vi "Functions_Load All.vi"(0 "scripts manager in":refnum<class "scripts manager.lvclass">, 5 "Function Path":path, 7 "Output Terminal":refnum<class "Output Terminal.lvclass">, 9 "RT Variables":refnum<class "RT Variables.lvclass">, 11 "error in (no error)":errorcluster) -> (4 "scripts manager out":refnum<class "scripts manager.lvclass">, 15 "error out":errorcluster)   [LabVIEW 2019, in "LSL.lvlib" / "scripts manager.lvclass"]
uses:
  scripts manager.lvclass
  output terminal/Base/Output Terminal.lvclass
  variables/RT Variables/RT Variables.lvclass
  scripts manager.lvclass/scripts manager.ctl
  functions/functionsbase/functionbase.lvclass
  functions/functionsbase/functionbase.lvclass/functionbase.ctl
  functions/functionsbase/properties/Write Output Terminal.vi
  functions/functionsbase/properties/Write RT Variables.vi
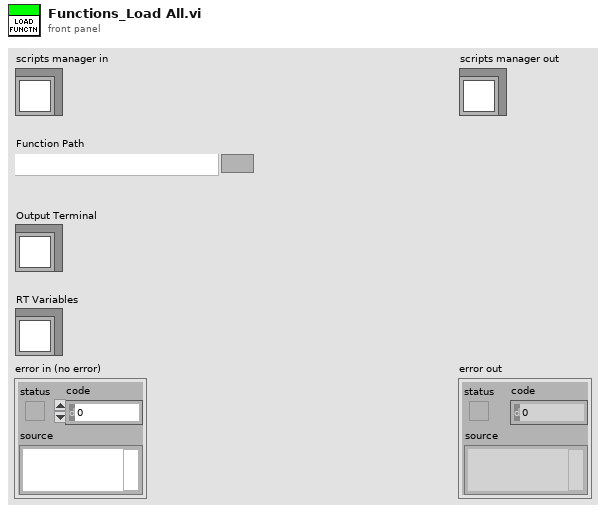
[diagram p1: front panel]
types:
  T1 = typedef "Scan Syntax Format.ctl" = cluster{"Format String":string, "Variable#":i32, "Variables Name":string[]}
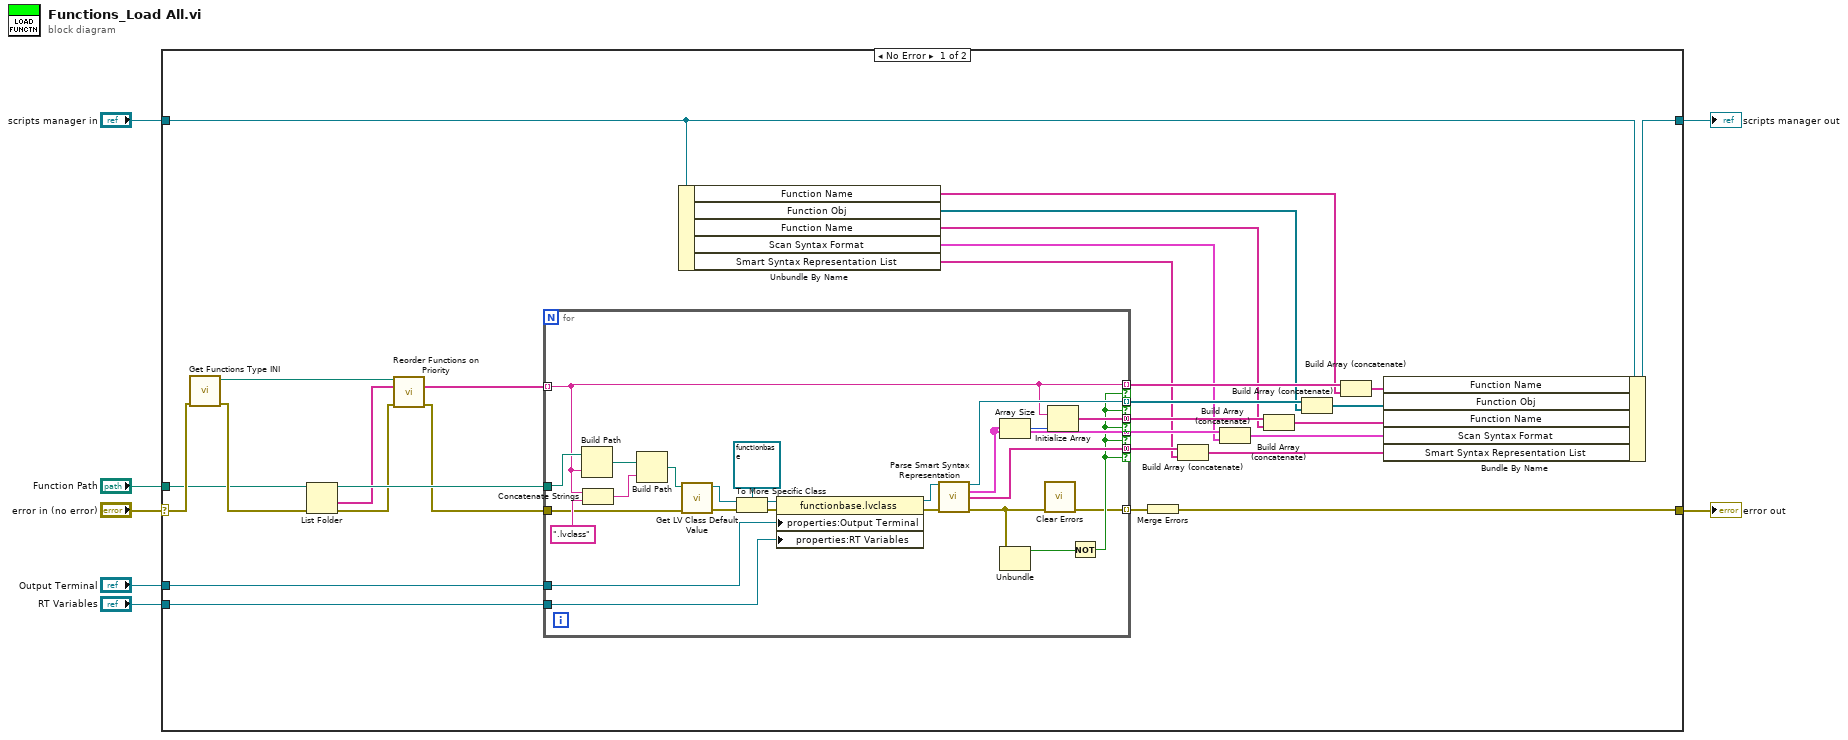
[diagram p0: block diagram]
diagram:
  n1 = case shown="No Error" "error in (no error)" {
    selector: "error in (no error)" -> [w22 w64]
    tunnel: [w31 w64] -> w6
    tunnel: [w32 w63] -> w4
    tunnel: "scripts manager in" -> [w19 w63]
    tunnel: "Output Terminal" -> [w28 _]
    tunnel: "RT Variables" -> [w27 _]
    tunnel: "Function Path" -> [w8 _]
    frame No Error {
      n2 = call "Get Functions Type INI.vi"("error in"=w22) -> ("error out"=w21:errorcluster, "Function Config INI"=w20:path)  [unwired: 9 in]
      n3 = List Folder(path=w8, error in=w21) -> (path out=w37:path, folder names=w23:string[], error out=w26:errorcluster)  [unwired: 2 in, 1 out]
      n4 = call "Reorder Functions on Priority.vi"("config path"=w20, "Function List"=w23, "error in (no error)"=w26) -> ("Function List out"=w24:string[], "error out"=w25:errorcluster)  [unwired: 11 in]
      n5 = for {
        tunnel: w25 -> [w57]
        tunnel: w24 -> [w48] mode=indexing
        tunnel: w37 -> [w62]
        tunnel: [w38] -> w36 mode=indexing
        tunnel: [w51] -> w29 mode=indexing if=w45
        tunnel: [w48] -> w30 mode=indexing if=w45
        tunnel: [w50] -> w35 mode=concatenating if=w45
        tunnel: [w47] -> w33 mode=concatenating if=w45
        tunnel: [w46] -> w34 mode=concatenating if=w45
        tunnel: w28 -> [w40]
        tunnel: w27 -> [w39]
        n6 = Build Path(base path=w62, name or relative path=w48) -> (appended path=w61:path)
        n7 = Concatenate Strings(w48, ".lvclass" ("string")) -> (w59:string)
        n8 = Build Path(base path=w61, name or relative path=w59) -> (appended path=w58:path)
        n9 = call <vilib>:"Get LV Class Default Value.vi"("error in (no error)"=w57, "class path"=w58) -> ("error out"=w56:errorcluster, "object"=w55:refnum<class>)  [unwired: 8 in]
        n10 = To More Specific Class(target class=refnum<class "functionbase.lvclass"> refnum ("functionbase.lvclass"), reference=w55, error in=w56) -> (specific class reference=w42:refnum<class "functionbase.lvclass">, error out=w44:errorcluster)
        n11 = property class="functionbase.lvclass"(reference=w42, error in=w44, "properties:Output Terminal"=w40, "properties:RT Variables"=w39) -> (reference out=w41:refnum<class "functionbase.lvclass">, error out=w43:errorcluster)
        n12 = call-dynamic "Parse Smart Syntax Representation.vi"("functionbase in"=w41, "error in (no error)"=w43) -> ("functionbase out"=w51:refnum<class "functionbase.lvclass">, "Scan Syntax List"=w50:T1[], "Smart Syntax Representation List"=w46:string[], "error out"=w52:errorcluster)  [unwired: 10 in]
        n13 = Array Size(array=w50) -> (size(s)=w49:i32)
        n14 = Unbundle(w52) -> ("status"=w53:bool)  [unwired: 2 out]
        n15 = call <vilib>:"Clear Errors.vi"("error in (no error)"=w52) -> ("error out"=w38:errorcluster)  [unwired: 5 in, 1 out]
        n16 = Initialize Array(w48, w49) -> (w47:string[])
        n17 = Not(x=w53) -> (.not. x?=w45:bool)
      }
      n18 = Unbundle By Name(w19) -> ("Function Name"=w17:string[], "Function Obj"=w15:refnum<class "functionbase.lvclass">[], "Function Name"=w13:string[], "Scan Syntax Format"=w11:T1[], "Smart Syntax Representation List"=w9:string[])
      n19 = Merge Errors(w36) -> (w31:errorcluster)
      n20 = Build Array (concatenate)(w34, w9) -> (w10:string[])
      n21 = Build Array (concatenate)(w35, w11) -> (w12:T1[])
      n22 = Build Array (concatenate)(w33, w13) -> (w14:string[])
      n23 = Build Array (concatenate)(w29, w15) -> (w16:refnum<class "functionbase.lvclass">[])
      n24 = Build Array (concatenate)(w30, w17) -> (w18:string[])
      n25 = Bundle By Name(cluster=w19, "Function Name"=w18, "Function Obj"=w16, "Function Name"=w14, "Scan Syntax Format"=w12, "Smart Syntax Representation List"=w10) -> (w32:refnum<class "scripts manager.lvclass">)
    }
    frame Error {
    }
  }
  "error out" <- w6
  "scripts manager out" <- w4
